vi "Switch Heater Status (Set).vi"(6 "ISOBUS address":T4=-1 caption="ISOBUS address (-1)", 8 "error in":errorcluster, 10 "Switch Heater Status":T1, 11 "Mercury Reference In":T5) -> (0 "error out":errorcluster, 2 "Response":T2, 3 "Mercury Reference Out":T5, 4 "Valid?":T3)   [LabVIEW 2015, in "Mercury iXX.lvlib" / "Magnet.lvlib"]
doc: "Set the switch heater status if Current = Persistant Current."
uses:
  Magnet.lvlib
  Controls/Mercury Reference.ctl
  Controls/Comms Transport Layer.ctl
  Private/Controls/Query Dynamic Reference.ctl
  Controls/ISOBus Address.ctl
  Controls/Is Valid LED.ctl
  Controls/Response String.ctl
  Controls/Switch Heater.ctl
  Private/Controls/Command Verbs.ctl
  Mercury iXX.lvlib
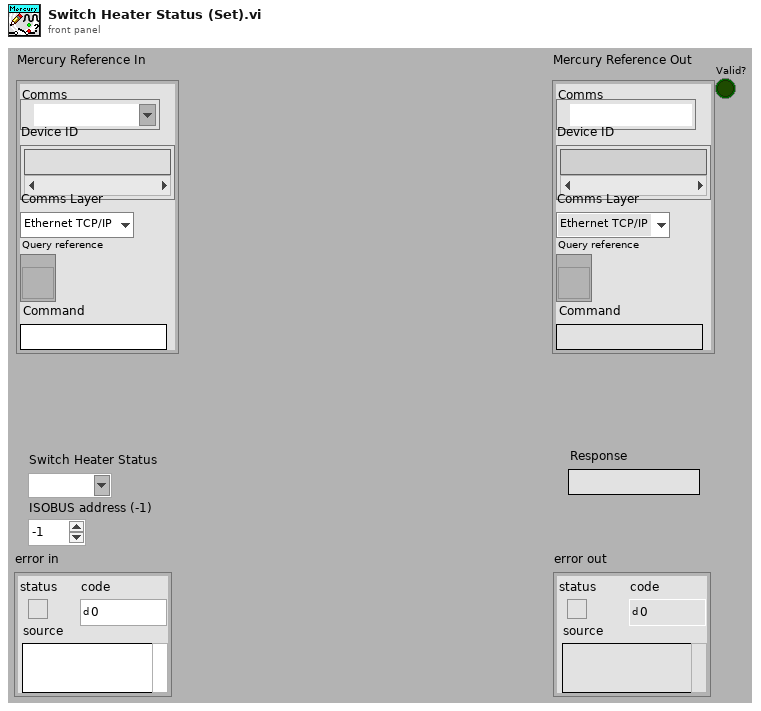
[diagram p1: front panel]
types:
  T1 = typedef "Mercury iXX.lvlib/Magnet.lvlib/Switch Heater.ctl" = string
  T2 = typedef "Mercury iXX.lvlib/Response String.ctl" = string
  T3 = typedef "Mercury iXX.lvlib/Is Valid LED.ctl" = bool
  T4 = typedef "Mercury iXX.lvlib/ISOBus Address.ctl" = i32
  T5 = typedef "Mercury iXX.lvlib/Mercury Reference.ctl" = cluster{"Comms":refnum<visa-resource-name>, "Device ID":string[], "Comms Layer":T6, "Command":string, "Query reference":T7}
  T6 = typedef "Mercury iXX.lvlib/Comms Transport Layer.ctl" = enum16{"Ethernet TCP/IP", "USB", "ISOBus - RS-232", "GPIB"}
  T7 = typedef "Mercury iXX.lvlib/Query Dynamic Reference.ctl" = refnum<vi>
  T8 = typedef "Mercury iXX.lvlib/Command Verbs.ctl" = string
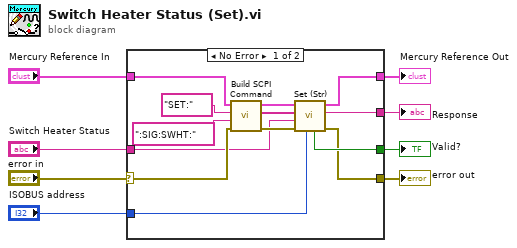
[diagram p0: block diagram]
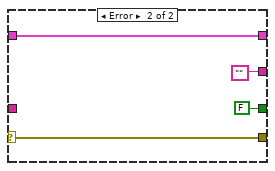
[diagram p2: hidden frame]
diagram:
  n1 = case shown="No Error" "error in" {
    selector: "error in" -> [w10 w24]
    tunnel: "ISOBUS address" -> [w21 _]
    tunnel: [w20 T3 FALSE ("Valid?")] -> w2
    tunnel: [w19 w25] -> w4
    tunnel: [w18 w24] -> w1
    tunnel: [w17 ""] -> w3
    tunnel: "Switch Heater Status" -> [w9 _]
    tunnel: "Mercury Reference In" -> [w14 w25]
    frame No Error {
      n2 = call "Build SCPI Command.vi"("error in"=w10, "Noun(s)"=":SIG:SWHT:" ("Command"), "Verb"=T8 "SET:", "Mercury Reference In"=w14) -> ("error out"=w12:errorcluster, "SCPI Message(s)"=w11:string[], "Mercury Reference Out"=w13:T5)  [unwired: 5 out]
      n3 = call "Set (Str).vi"("ISOBUS address"=w21, "error in"=w12, "Command Value (Str)"=w9, "SCPI Message(s)"=w11, "Mercury Reference In"=w13) -> ("error out"=w18:errorcluster, "Response"=w17:T2, "Mercury Reference Out"=w19:T5, "Valid?"=w20:T3)  [unwired: 1 in, 2 out]
    }
    frame Error {
    }
  }
  "Mercury Reference Out" <- w4
  "Valid?" <- w2
  "error out" <- w1
  "Response" <- w3
